vi "Set Enum String Value__ogtk.vi"(8 "error in (no error)":errorcluster, 9 "String Value":string, 10 "Default Enum Value":variant) -> (0 "error out":errorcluster, 2 "Enum":variant)   [LabVIEW 2019]
doc: "Sets an enum's integer value to the position within the enum's strings matching the <B>String Value</B> input. Returns<B> Default Enum Value</B> if an error occurs."
panel:
  # "[OpenG VI Tags] ***Do Not Remove***"
  # "Set Enum String Value.vi\n\nSets an enum's integer value to the position within the enum's strings matching \n\nPlease visit http://www.OpenG.org to learn about the\nOpen Source LabVIEW software movement.\n\nNOTICE -- YOU MUST LEAVE THIS NOTICE IN PLACE.  PER THE TERMS OF THE LICENSE BELOW, YOU MAY SUBLICENSE THIS SOFTWARE \nIN ANY WAY THAT DOES NOT CONFLICT WITH THIS LICENSE.\n\n### BSD License (http://www.opensource.org/licenses/bsd-license.php) Begin ###\n \nCopyright (c) 2002, Jean-Pierre Drolet <drolet_jp@hotmail.com>\nCopyright (c) 2002-2006, Jim Kring <jim@jimkring.com>\n\nAll rights reserved.\n\nRedistribution and use in source and binary forms, with or without modification, are permitted provided that the following conditions are met:\n\n    * Redistributions of source code must retain the above copyright notice, this list of conditions and the following disclaimer.\n    * Redistributions in binary form must reproduce the above copyright notice, this list of conditions and the following disclaimer in the \n       documentation and/or other materials provided with the distribution.\n    * Neither the name of SciWare, James Kring, Inc., nor the names of its contributors may be used to endorse or promote products derived \n       from this software without specific prior written permission.\n\nTHIS SOFTWARE IS PROVIDED BY THE COPYRIGHT HOLDERS AND CONTRIBUTORS \"AS IS\" AND ANY EXPRESS OR IMPLIED WARRANTIES, \nINCLUDING, BUT NOT LIMITED TO, THE IMPLIED WARRANTIES OF MERCHANTABILITY AND FITNESS FOR A PARTICULAR PURPOSE ARE \nDISCLAIMED. IN NO EVENT SHALL THE COPYRIGHT OWNER OR CONTRIBUTORS BE LIABLE FOR ANY DIRECT, INDIRECT, INCIDENTAL,\n SPECIAL, EXEMPLARY, OR CONSEQUENTIAL DAMAGES (INCLUDING, BUT NOT LIMITED TO, PROCUREMENT OF SUBSTITUTE GOODS OR \nSERVICES; LOSS OF USE, DATA, OR PROFITS; OR BUSINESS INTERRUPTION) HOWEVER CAUSED AND ON ANY THEORY OF LIABILITY, \nWHETHER IN CONTRACT, STRICT LIABILITY, OR TORT (INCLUDING NEGLIGENCE OR OTHERWISE) ARISING IN ANY WAY OUT OF THE USE \nOF THIS SOFTWARE, EVEN IF ADVISED OF THE POSSIBILITY OF SUCH DAMAGE.\n\n### BSD License End ###"
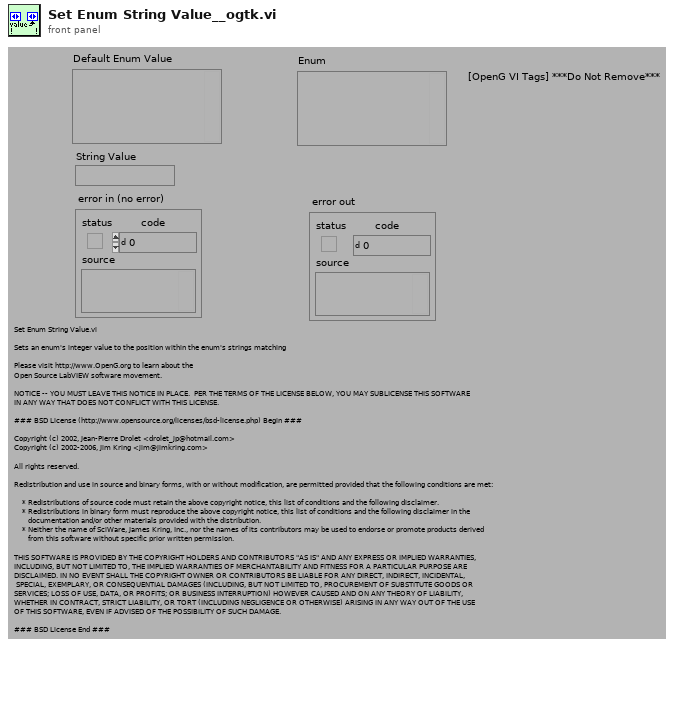
[diagram p1: front panel]
types:
  T1 = typedef "Type Descriptor Header__ogtk.ctl" = cluster{"length":u16, "private":u8, "type":T2, "# elements":u16}
  T2 = typedef "Type Descriptor Enumeration__ogtk.ctl" = enum8{"<Null>", "I8", "I16", "I32", "I64", "U8", "U16", "U32", "U64", "SGL", "DBL", "EXT", "CSG", "CDB", "CXT", "0x0F", "0x10", "0x11", "0x12", "0x13", "0x14", "Enum U8", "Enum U16", "Enum U32", "Enum U64", "SGL PQ", "DBL PQ", "EXT PQ", "CSG PQ", "CDB PQ", "CXT PQ", "0x1F", "0x20", "Boolean", "0x22", "0x23", "0x24", "0x25", "0x26", "0x27", "0x28", "0x29", "0x2A", "0x2B", "0x2C", "0x2D", "0x2E", "0x2F", "String", "0x31", "Path", "Pict", "0x34", "0x35", "0x36", "DAQ", "0x38", "0x39", "0x3A", "0x3B", "0x3C", "0x3D", "0x3E", "0x3F", "Array", "0x41", "0x42", "0x43", "0x44", "0x45", "0x46", "0x47", "0x48", "0x49", "0x4A", "0x4B", "0x4C", "0x4D", "0x4E", "0x4F", "Cluster", "0x51", "0x52", "Variant", "Waveform", "0x55", "0x56", "0x57", "0x58", "0x59", "0x5A", "0x5B", "0x5C", "0x5D", "0x5E", "Fixed Point", "0x60", "0x61", "0x62", "0x63", "0x64", "0x65", "0x66", "0x67", "0x68", "0x69", "0x6A", "0x6B", "0x6C", "0x6D", "0x6E", "0x6F", "Refnum", "0x71", "0x72", "Set Collection", "Map Collection"}
  T3 = typedef "Type Descriptor__ogtk.ctl" = i16[]
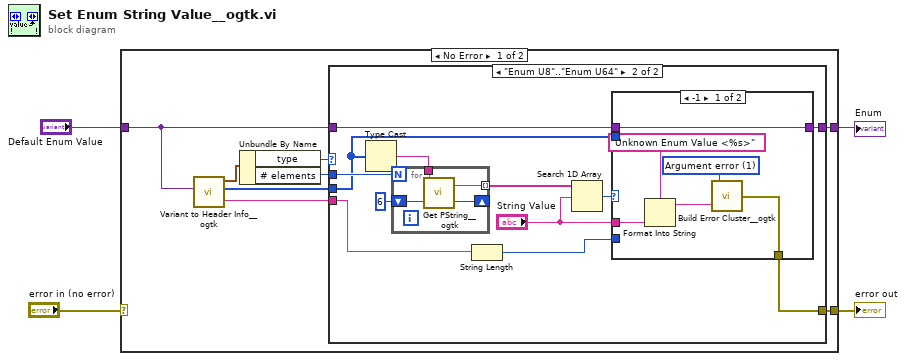
[diagram p0: block diagram]
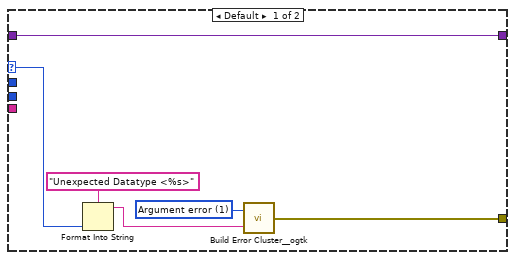
[diagram p2: hidden frame]
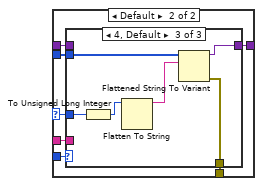
[diagram p3: hidden frame]
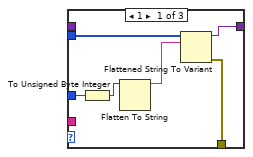
[diagram p4: hidden frame]
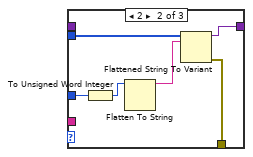
[diagram p5: hidden frame]
diagram:
  n1 = case shown="No Error" "error in (no error)" {
    selector: "error in (no error)" -> [_ w67]
    tunnel: [w12 w67] -> w4
    tunnel: [w6 w66] -> w2
    tunnel: "Default Enum Value" -> [w5 w66]
    frame No Error {
      n2 = call "Variant to Header Info__ogtk.vi"("Variant"=w5) -> ("Type Descriptor Header"=w11:T1, "Type Descriptor"=w9:T3, "data string"=w8:string)  [unwired: 3 in]
      n3 = Unbundle By Name(w11) -> ("type"=w10:T2, "# elements"=w7:u16)
      n4 = case shown="\"Enum U8\"..\"Enum U64\"" w10 {
        selector: w10 -> [w15 _]
        tunnel: [w18 w21] -> w12
        tunnel: w9 -> [_ w22]
        tunnel: w8 -> [_ w25]
        tunnel: w7 -> [_ w28]
        tunnel: [w16 w23] -> w6
        tunnel: w5 -> [w16 w24]
        frame Default {
          w17 = 1 items=["No error", "Argument error", "Memory is full", "Out of zone", "End of file", "File already open", "Generic file I/O error", "File not found", "File permission error", "Disk is full", "Duplicate path", "Too many files open", "System feature not enabled", "Resource file not found", "Cannot add resource", "Resource not found", "Image not found", "Image memory error", "Pen does not exist", "Config type invalid", "Config token not found", "Config parse error", "Config memory error", "Bad external code format", "Bad external code offset", "External code not present", "Null window", "Destroy window error", "Null menu", "Print aborted", "Bad print record", "Print driver error", "Windows error during printing", "Memory error during printing", "Print dialog error", "Generic print error", "Invalid device refnum", "Device not found", "Device parameter error", "Device unit error", "Cannot open device", "Device call aborted", "Generic error", "Cancelled by user", "Object ID too low", "Object ID too high", "Object not in heap", "Unknown heap", "Unknown object (invalid DefProc)", "Unknown object (DefProc not in table)", "Message out of range", "Invalid (null) method", "Unknown message", "Manager call not supported", "Bad address", "Network operation in progress", "Network operation timed out", "Connection is busy", "Network attribute not supported", "Network error", "Address in use", "System out of memory", "Connection aborted", "Connection refused", "Not connected", "Already connected", "Connection closed", "Initialization error (interapplication manager)", "Bad occurrence", "Wait on unbound occurrence handler", "Occurrence queue overflow", "Datalog type conflict", "Unused", "Unrecognized type (interapplication manager)", "Memory corrupt", "Failed to make temporary DLL", "Old CIN version", "Drag socket not found", "Failed to load drop-object", "Failed to register OLE object", "Failed to release OLE object", "Format specifier type mismatch", "Unknown format specifier", "Too few format specifiers", "Too many format specifiers", "Scan failed", "Newer CIN version", "Error converting to variant", "Runtime menu error", "Password tampered", "Variant attribute not found", "Incompatible variant data type", "Event data is not available", "Event Store is not present", "Occurrence is not found", "Event Queue is not created", "Event info is not available", "Refnum passed is NULL", "Error retrieving Class GUID", "Error retrieving CoClass GUID", "Error retrieving TypeLib GUID.", "Bad built application magic bytes.", "Specific driver is different from the specific driver associated with the Logical Name.", "There is no session opened to the class driver.", "Max Error", "MAX - Error with config objects", "MAX - Error loading configuration", "MAX - Group not supported"]
          n5 = Format Into String(format string="Unexpected Datatype <%s>" ("Format String"), w15) -> (resulting string=w13:string)  [unwired: 2 in, 1 out]
          n6 = call "Build Error Cluster__ogtk.vi"("String to Prepend to source (\"\")"=w13, "code"=w17) -> ("error out"=w18:errorcluster)
        }
        frame "Enum U8".."Enum U64" {
          n7 = Type Cast(x=w22) -> (*(type *) &x=w27:string)  [unwired: 1 in]
          n8 = for {
            N: w28 -> [_]
            tunnel: w27 -> [w63]
            shift-right: [w64] -> _
            shift-left: 6 -> [w65]
            tunnel: [w62] -> w26 mode=indexing
            n9 = call "Get PString__ogtk.vi"("offset (0)"=w65, "String"=w63) -> ("offset past PString"=w64:i32, "PString"=w62:string)
          }
          n10 = String Length(string=w25) -> (length=w29:i32)
          n11 = Search 1D Array(1D array=w26, element="String Value") -> (index of element=w19:i32)  [unwired: 1 in]
          n12 = case shown="-1" w19 {
            selector: w19 -> [_ w37]
            tunnel: w29 -> [_ w43]
            tunnel: w24 -> [w36 w42]
            tunnel: [w36 w41] -> w23
            tunnel: w22 -> [_ w40]
            tunnel: [w31 w39] -> w21
            tunnel: "String Value" -> [w32 w38]
            frame -1 {
              w35 = 1 items=["No error", "Argument error", "Memory is full", "Out of zone", "End of file", "File already open", "Generic file I/O error", "File not found", "File permission error", "Disk is full", "Duplicate path", "Too many files open", "System feature not enabled", "Resource file not found", "Cannot add resource", "Resource not found", "Image not found", "Image memory error", "Pen does not exist", "Config type invalid", "Config token not found", "Config parse error", "Config memory error", "Bad external code format", "Bad external code offset", "External code not present", "Null window", "Destroy window error", "Null menu", "Print aborted", "Bad print record", "Print driver error", "Windows error during printing", "Memory error during printing", "Print dialog error", "Generic print error", "Invalid device refnum", "Device not found", "Device parameter error", "Device unit error", "Cannot open device", "Device call aborted", "Generic error", "Cancelled by user", "Object ID too low", "Object ID too high", "Object not in heap", "Unknown heap", "Unknown object (invalid DefProc)", "Unknown object (DefProc not in table)", "Message out of range", "Invalid (null) method", "Unknown message", "Manager call not supported", "Bad address", "Network operation in progress", "Network operation timed out", "Connection is busy", "Network attribute not supported", "Network error", "Address in use", "System out of memory", "Connection aborted", "Connection refused", "Not connected", "Already connected", "Connection closed", "Initialization error (interapplication manager)", "Bad occurrence", "Wait on unbound occurrence handler", "Occurrence queue overflow", "Datalog type conflict", "Unused", "Unrecognized type (interapplication manager)", "Memory corrupt", "Failed to make temporary DLL", "Old CIN version", "Drag socket not found", "Failed to load drop-object", "Failed to register OLE object", "Failed to release OLE object", "Format specifier type mismatch", "Unknown format specifier", "Too few format specifiers", "Too many format specifiers", "Scan failed", "Newer CIN version", "Error converting to variant", "Runtime menu error", "Password tampered", "Variant attribute not found", "Incompatible variant data type", "Event data is not available", "Event Store is not present", "Occurrence is not found", "Event Queue is not created", "Event info is not available", "Refnum passed is NULL", "Error retrieving Class GUID", "Error retrieving CoClass GUID", "Error retrieving TypeLib GUID.", "Bad built application magic bytes.", "Specific driver is different from the specific driver associated with the Logical Name.", "There is no session opened to the class driver.", "Max Error", "MAX - Error with config objects", "MAX - Error loading configuration", "MAX - Group not supported"]
              n13 = Format Into String(format string="Unknown Enum Value <%s>" ("Format String"), w32) -> (resulting string=w34:string)  [unwired: 2 in, 1 out]
              n14 = call "Build Error Cluster__ogtk.vi"("String to Prepend to source (\"\")"=w34, "code"=w35) -> ("error out"=w31:errorcluster)
            }
            frame Default {
              n15 = case shown="4, Default" w43 {
                tunnel: w37 -> [w49 w55 w61]
                tunnel: w42 -> [_ _ _]
                tunnel: [w45 w51 w57] -> w41
                tunnel: w40 -> [w47 w53 w59]
                tunnel: [w44 w50 w56] -> w39
                tunnel: w38 -> [_ _ _]
                frame 1 {
                  n16 = To Unsigned Byte Integer(number=w49) -> (unsigned 8bit integer=w48:u8)
                  n17 = Flatten To String(anything=w48) -> (data string=w46:string)  [unwired: 3 in, 2 out]
                  n18 = Flattened String To Variant(6:w46, 7:w47) -> (0:w44:errorcluster, 3:w45:variant)  [unwired: 1 in]
                }
                frame 2 {
                  n19 = To Unsigned Word Integer(number=w55) -> (unsigned 16bit integer=w54:u16)
                  n20 = Flatten To String(anything=w54) -> (data string=w52:string)  [unwired: 3 in, 2 out]
                  n21 = Flattened String To Variant(6:w52, 7:w53) -> (0:w50:errorcluster, 3:w51:variant)  [unwired: 1 in]
                }
                frame 4, Default {
                  n22 = To Unsigned Long Integer(number=w61) -> (unsigned 32bit integer=w60:u32)
                  n23 = Flatten To String(anything=w60) -> (data string=w58:string)  [unwired: 3 in, 2 out]
                  n24 = Flattened String To Variant(6:w58, 7:w59) -> (0:w56:errorcluster, 3:w57:variant)  [unwired: 1 in]
                }
              }
            }
          }
        }
      }
    }
    frame Error {
    }
  }
  "error out" <- w4
  "Enum" <- w2
